vi "empty string subs.vi"(8 "Ctl Refnum":refnum<vi>, 10 "String":string) -> (2 "Nova String":string)   [LabVIEW 2019]
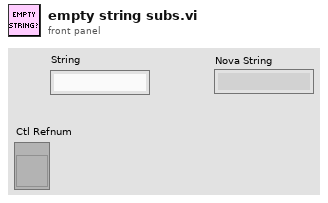
[diagram p1: front panel]
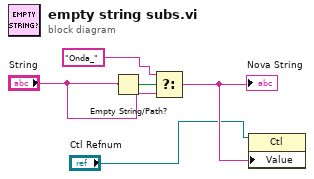
[diagram p0: block diagram]
diagram:
  n1 = Empty String/Path?(string/path="String") -> (empty?=w5:bool)
  n2 = Select(t="Onda_" ("String"), s=w5, f="String") -> (s? t:f=w2:string)
  "Nova String" <- w2
  n3 = property class="Ctl"(reference="Ctl Refnum", "Value"=w2) -> ()  [unwired: 1 in, 2 out]
